vi "1_PLANTILLA.vi"() -> ()   [LabVIEW 2019]
panel:
  out "String_ind":string
  in  "String_ctrl":string
  out "Num_ind":dbl
  in  "Num_ctrl":dbl
  in  "stop":bool
  out "N_ITERACION":i32
  in  "INTERRUPTOR":bool
  out "LED":bool
  out "SENOIDE":dbl[](graph)
  # "PLANTILLA TELEMÁTICA"
  # "TERMINALES"
  # "CONTROL"
  # "INDICADOR"
  # "(C) 2020"
  # "J.LUIS PÉREZ DEL VAL"
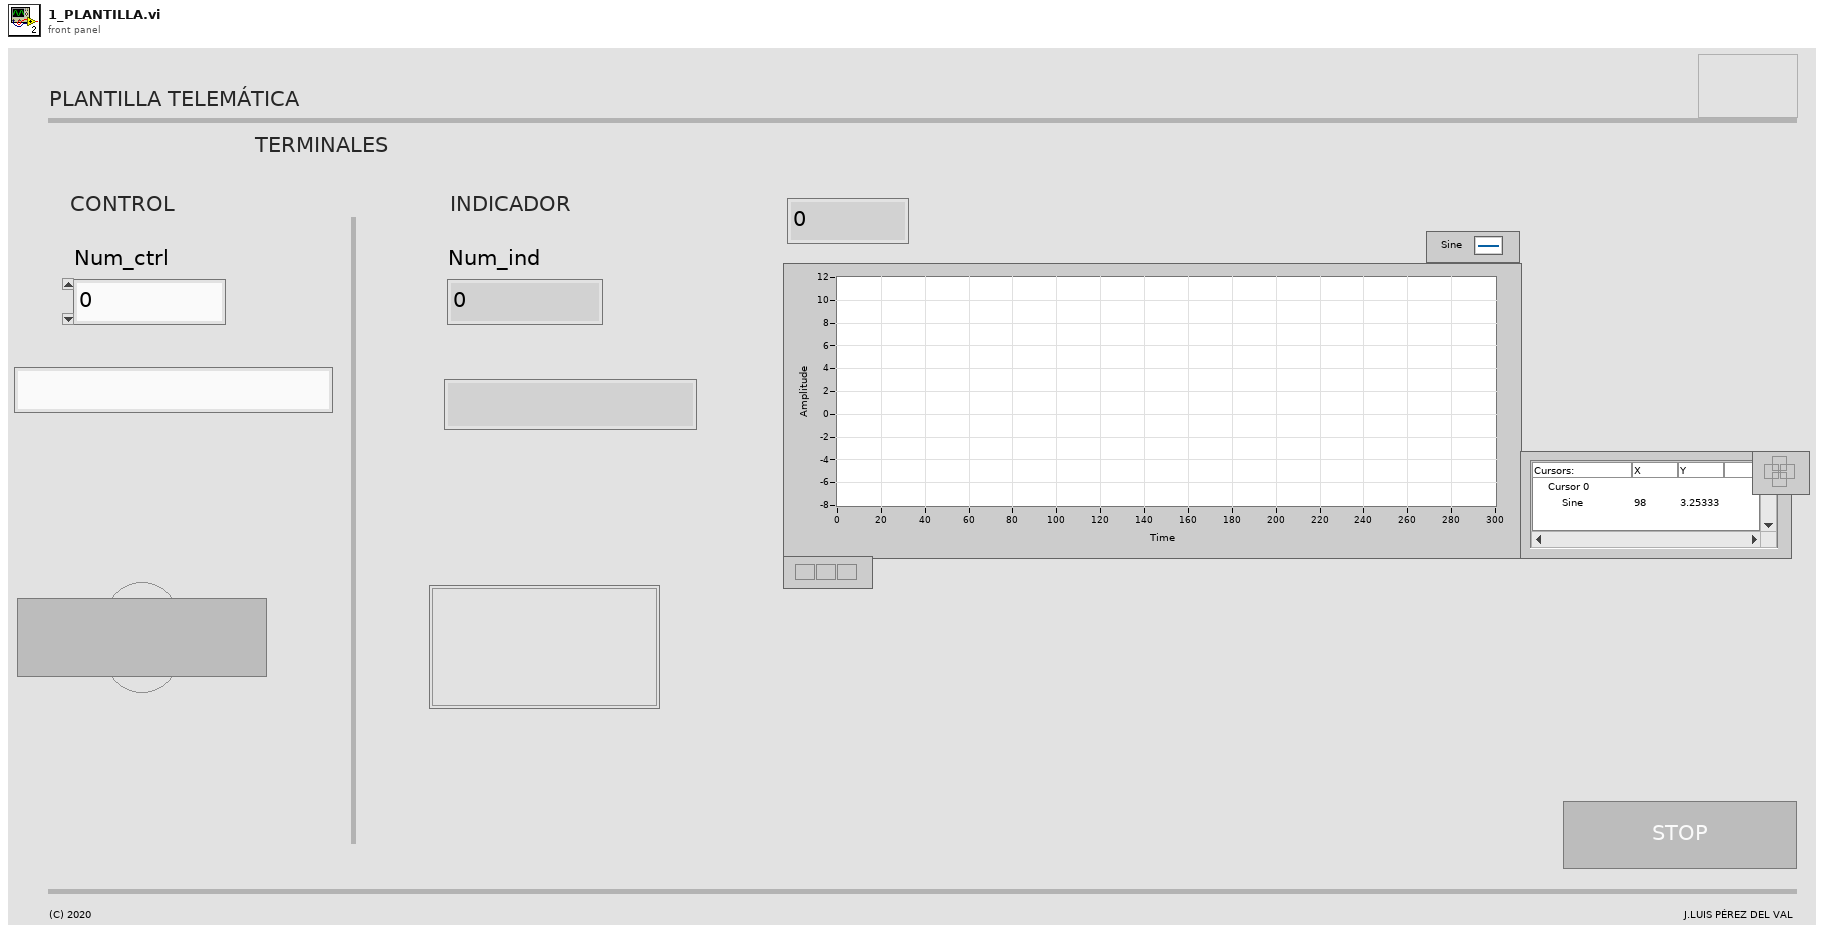
[diagram p1: front panel]
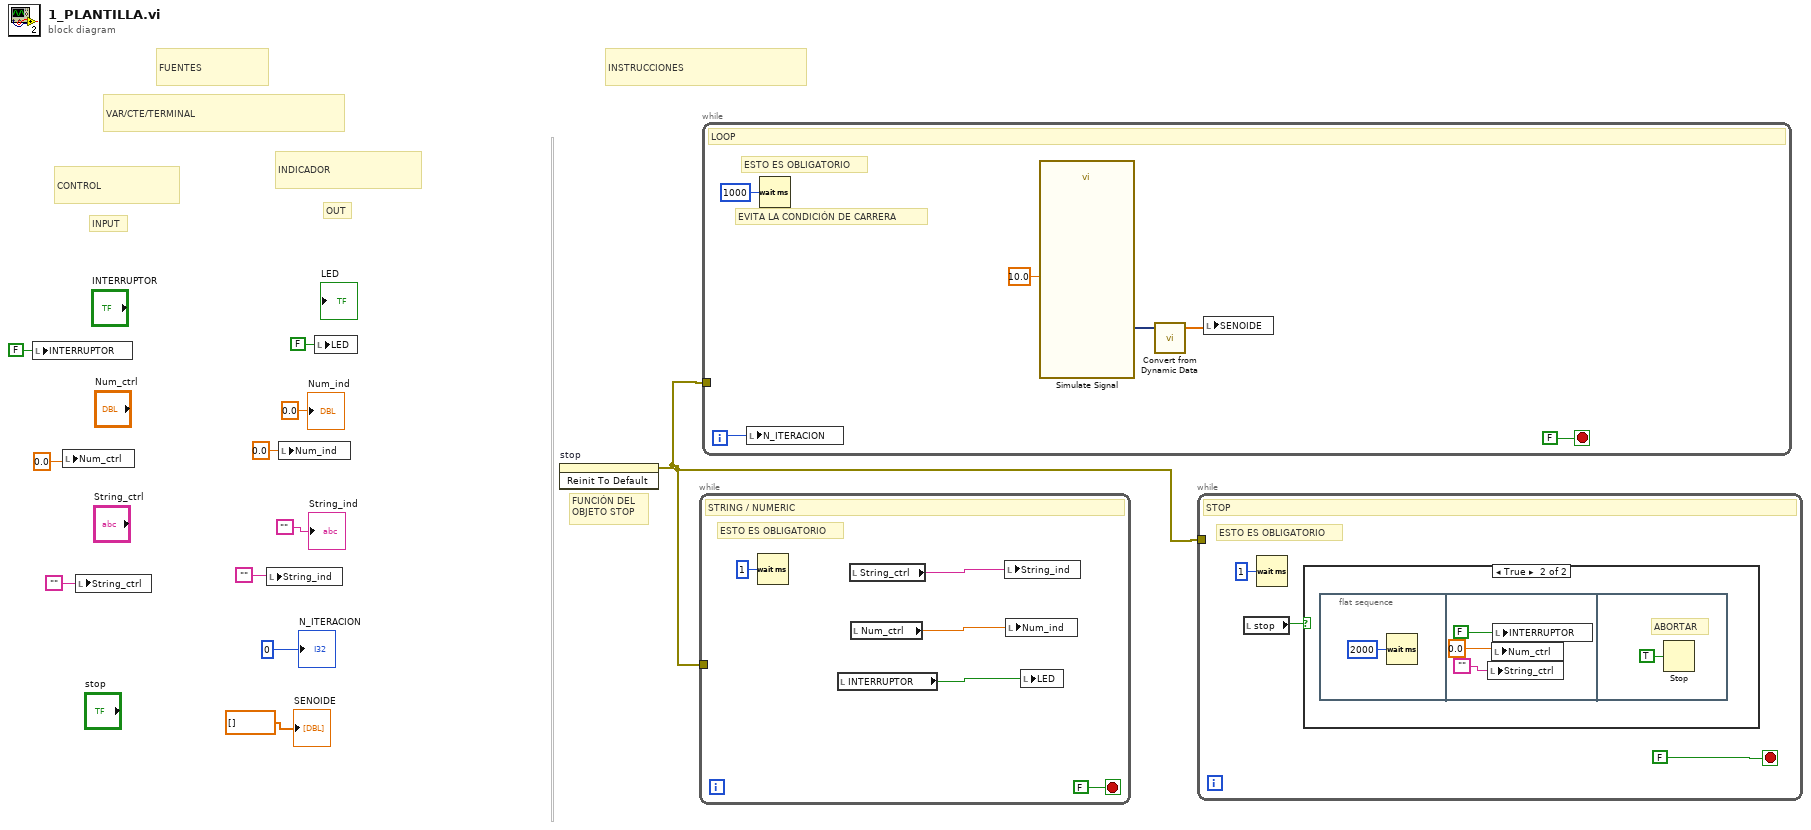
[diagram p0: block diagram]
diagram:
  # "FUNCIÓN DEL\nOBJETO STOP"
  # "INSTRUCCIONES"
  # "OUT"
  # "INPUT"
  # "INDICADOR"
  # "CONTROL"
  # "VAR/CTE/TERMINAL"
  # "FUENTES"
  n1 = local write "INTERRUPTOR"(FALSE ("INTERRUPTOR")) -> ()
  n2 = local write "Num_ctrl"(0.0) -> ()
  n3 = local write "String_ctrl"("") -> ()
  n4 = local write "String_ind"("") -> ()
  n5 = local write "Num_ind"(0.0 ("Num_ind")) -> ()
  n6 = local write "LED"(FALSE ("LED")) -> ()
  n7 = invoke on="stop" class="Bool (strict)" method="Reinit To Default"() -> (error out=w1:errorcluster)  [unwired: 3 in, 2 out]
  n8 = while {
    tunnel: w1 -> [_]
    stop <- FALSE stop-if-true
    # "ESTO ES OBLIGATORIO"
    # "STRING / NUMERIC"
    n9 = Wait (ms)(milliseconds to wait=u32 1) -> ()  [unwired: 1 out]
    n10 = local read "INTERRUPTOR"() -> (w14:bool)
    n11 = local read "String_ctrl"() -> (w16:string)
    n12 = local read "Num_ctrl"() -> (w15:dbl)
    n13 = local write "String_ind"(w16) -> ()
    n14 = local write "Num_ind"(w15) -> ()
    n15 = local write "LED"(w14) -> ()
  }
  n16 = while {
    tunnel: w1 -> [_]
    i -> [w20]
    stop <- FALSE stop-if-true
    # "EVITA LA CONDICIÓN DE CARRERA"
    # "ESTO ES OBLIGATORIO"
    # "LOOP"
    n17 = local write "N_ITERACION"(w20) -> ()
    n18 = Wait (ms)(milliseconds to wait=u32 1000) -> ()  [unwired: 1 out]
    n19 = call "Simulate Signal"("Amplitude"=10.0) -> ("Sine"=w22:dynamicdata)  [unwired: 13 in, 1 out]
    n20 = call "Convert from Dynamic Data"("Dynamic Data Type"=w22) -> ("Array"=w21:dbl[])  [unwired: 3 in]
    n21 = local write "SENOIDE"(w21) -> ()
  }
  n22 = while {
    tunnel: w1 -> [_]
    stop <- FALSE stop-if-true
    # "ESTO ES OBLIGATORIO"
    # "STOP"
    n23 = local read "stop"() -> (w23:bool)
    n24 = Wait (ms)(milliseconds to wait=u32 1) -> ()  [unwired: 1 out]
    n25 = case shown="True" w23 {
      frame False {
      }
      frame True {
        n26 = flat-sequence {
          frame #0 {
            n27 = Wait (ms)(milliseconds to wait=u32 2000) -> ()  [unwired: 1 out]
          }
          frame #1 {
            n28 = local write "String_ctrl"("") -> ()
            n29 = local write "Num_ctrl"(0.0 ("Num_ind")) -> ()
            n30 = local write "INTERRUPTOR"(FALSE ("LED")) -> ()
          }
          frame #2 {
            # "ABORTAR"
            n31 = Stop(stop? (T)=TRUE) -> ()
          }
        }
      }
    }
  }
  "SENOIDE" <- dbl[] [] ("Waveform Graph")
  "N_ITERACION" <- 0 ("Numeric")
  "Num_ind" <- 0.0
  "String_ind" <- ""
